vi "Untitled 6.vi"() -> ()   [LabVIEW 2021]
panel:
  in  "stop":bool
  out "XY Graph":cluster{i32[], dbl[]}[](graph)
  in  "Установка":dbl
  out "I":dbl
  in  "dt":dbl
  out "Даткчик":dbl
  out "IprevErr":dbl
  in  "kp":dbl
  in  "ki":dbl
  in  "kd":dbl
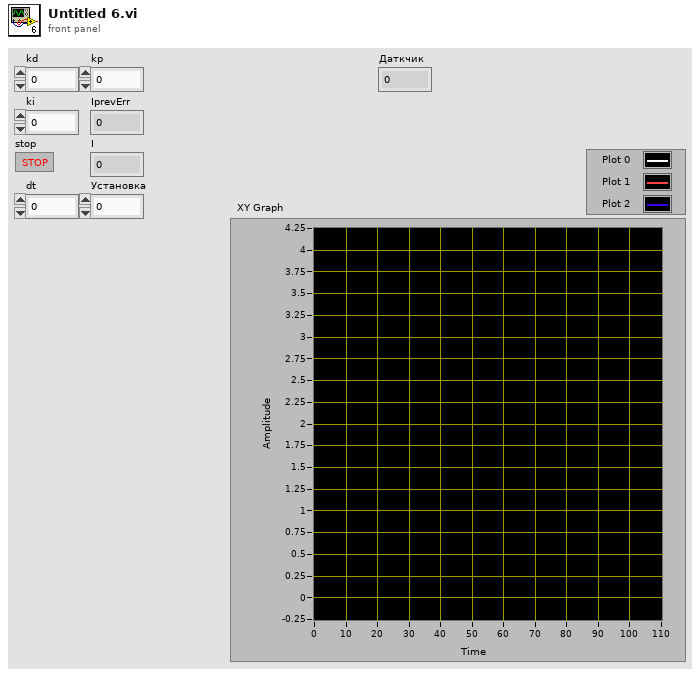
[diagram p1: front panel]
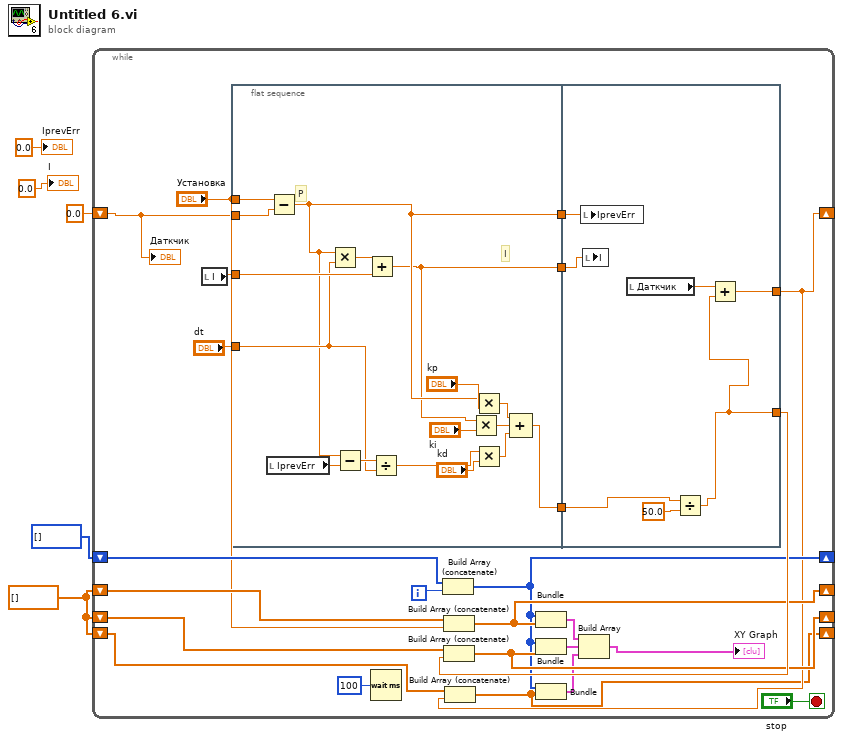
[diagram p0: block diagram]
diagram:
  w1 = dbl[] []
  n1 = while {
    shift-right: [w11] -> _
    shift-left: i32[] [] -> [w22]
    shift-right: [w15] -> _
    shift-left: w1 -> [w20]
    shift-right: [w7] -> _
    shift-left: 0.0 -> [w13]
    shift-right: [w16] -> _
    shift-left: w1 -> [w19]
    shift-right: [w6] -> _
    shift-left: w1 -> [w8]
    i -> [w23]
    stop <- "stop" stop-if-true
    n2 = local read "I"() -> (w28:dbl)
    n3 = flat-sequence {
      tunnel: "Установка" -> [w36]
      tunnel: w13 -> [w30]
      tunnel: w28 -> [w35]
      tunnel: "dt" -> [w34]
      tunnel: [w33] -> w26
      tunnel: [w32] -> w25
      tunnel: [w31] -> w24
      tunnel: w26 -> [w50]
      tunnel: w25 -> [w53]
      tunnel: w24 -> [w52]
      tunnel: [w47] -> w17
      tunnel: [w51] -> w7
      frame #0 {
        # "I"
        # "P"
        n4 = local read "IprevErr"() -> (w38:dbl)
        n5 = Subtract(x=w36, y=w30) -> (x-y=w32:dbl)
        n6 = Multiply(x=w32, y=w34) -> (x*y=w37:dbl)
        n7 = Subtract(x=w32, y=w38) -> (x-y=w39:dbl)
        n8 = Add(x=w37, y=w35) -> (x+y=w31:dbl)
        n9 = Divide(x=w39, y=w34) -> (x/y=w43:dbl)
        n10 = Multiply(x=w31, y="ki") -> (x*y=w41:dbl)
        n11 = Multiply(x=w32, y="kp") -> (x*y=w40:dbl)
        n12 = Multiply(x=w43, y="kd") -> (x*y=w42:dbl)
        n13 = Compound Arithmetic op=ADD(w40, w41, w42) -> (w33:dbl)
      }
      frame #1 {
        n14 = local write "IprevErr"(w53) -> ()
        n15 = local write "I"(w52) -> ()
        n16 = local read "Даткчик"() -> (w48:dbl)
        n17 = Divide(x=w50, y=50.0) -> (x/y=w47:dbl)
        n18 = Add(x=w48, y=w47) -> (x+y=w51:dbl)
      }
    }
    n19 = Wait (ms)(milliseconds to wait=u32 100) -> ()  [unwired: 1 out]
    n20 = Build Array (concatenate)(w22, w23) -> (w11:i32[])
    n21 = Build Array (concatenate)(w20, "Установка") -> (w15:dbl[])
    n22 = Build Array (concatenate)(w19, w17) -> (w16:dbl[])
    n23 = Build Array (concatenate)(w8, w7) -> (w6:dbl[])
    n24 = Bundle(w11, w15) -> (w29:cluster{i32[], dbl[]})  [unwired: 1 in]
    n25 = Bundle(w11, w16) -> (w10:cluster{i32[], dbl[]})  [unwired: 1 in]
    n26 = Bundle(w11, w6) -> (w9:cluster{i32[], dbl[]})  [unwired: 1 in]
    n27 = Build Array(w29, w10, w9) -> (→"XY Graph":cluster{i32[], dbl[]}[])
    "Даткчик" <- w13
  }
  "IprevErr" <- 0.0 ("IprevErr")
  "I" <- 0.0 ("IprevErr")
